vi "InterpretFSS.vi"(5 "FSS in":refnum<class "FlatSequence.lvclass">, 6 "error in":errorcluster, 9 "VI Interpreter in":refnum<class "VI Interpreter.lvclass">) -> (0 "error out":errorcluster, 3 "VI Interpreter out":refnum<class "VI Interpreter.lvclass">, 4 "FSS out":refnum<class "FlatSequence.lvclass">)   [LabVIEW 2014, in "VI Interpreter.lvclass"]
uses:
  VI Interpreter.lvclass
  FlatSequence/FlatSequence.lvclass
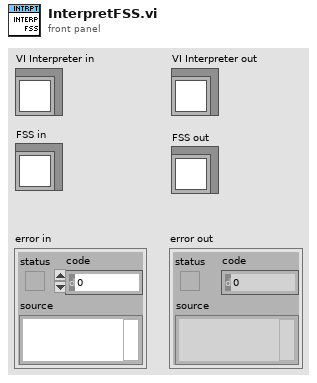
[diagram p1: front panel]
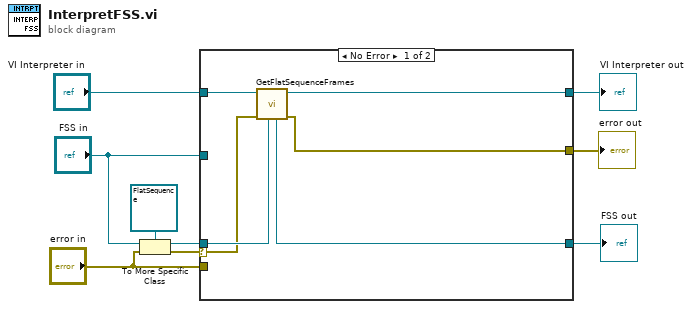
[diagram p0: block diagram]
diagram:
  n1 = To More Specific Class(target class=refnum<class "FlatSequence.lvclass"> refnum ("flat sequence"), reference="FSS in", error in="error in") -> (specific class reference=w5:refnum<class "FlatSequence.lvclass">, error out=w4:errorcluster)
  n2 = case shown="No Error" w4 {
    selector: w4 -> [w10 _]
    tunnel: "VI Interpreter in" -> [w15 w17]
    tunnel: [w11 w16] -> w8
    tunnel: [w14 w17] -> w7
    tunnel: [w12 w18] -> w6
    tunnel: w5 -> [w13 _]
    tunnel: "error in" -> [_ w18]
    tunnel: "FSS in" -> [_ w16]
    frame No Error {
      n3 = call "GetFlatSequenceFrames.vi"("FlatSequence in"=w13, "error in"=w10, "VI Interpreter in"=w15) -> ("error out"=w12:errorcluster, "VI Interpreter out"=w14:refnum<class "VI Interpreter.lvclass">, "FlatSequence out"=w11:refnum<class "FlatSequence.lvclass">)  [unwired: 4 in]
    }
    frame Error {
    }
  }
  "error out" <- w6
  "VI Interpreter out" <- w7
  "FSS out" <- w8
